vi "computername.vi"(2 "error in (no error)":errorcluster, 3 "value":string="ComputerName", 4 "subkey":string="System\\CurrentControlSet\\Control\\ComputerName\\ComputerName", 5 "root key (HKEY_LOCAL_MACHINE)":T1=enum."HKEY_LOCAL_MACHINE") -> (0 "error out":errorcluster, 1 "String/Binary data":string)   [LabVIEW 2018]
doc: "This example program uses the Registry VIs in LabVIEW to access the Windows registry and obtain the computer name."
uses:
  <vilib>/registry/registry.llb/Registry RtKey.ctl
  <vilib>/registry/registry.llb/Read Registry Value Simple STR.vi
panel:
  # "This example program uses the Registry VIs in LabVIEW to access the Windows registry and obtain the computer name.\n\nTo Run the program, click on the Run arrow. The computer name will be shown in the 'String/Binary data' string indicator."
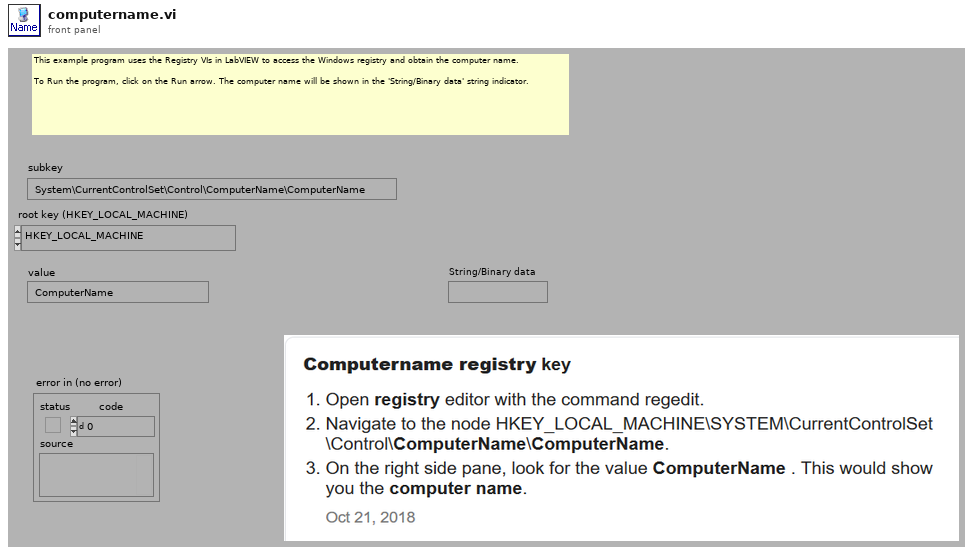
[diagram p1: front panel]
types:
  T1 = typedef "Registry RtKey.ctl" = enum32{"HKEY_CLASSES_ROOT", "HKEY_CURRENT_USER", "HKEY_LOCAL_MACHINE", "HKEY_USERS", "HKEY_PERFORMANCE_DATA", "HKEY_CURRENT_CONFIG", "HKEY_DYN_DATA"}
  T2 = typedef "Registry refnum.ctl" = refnum<k1>
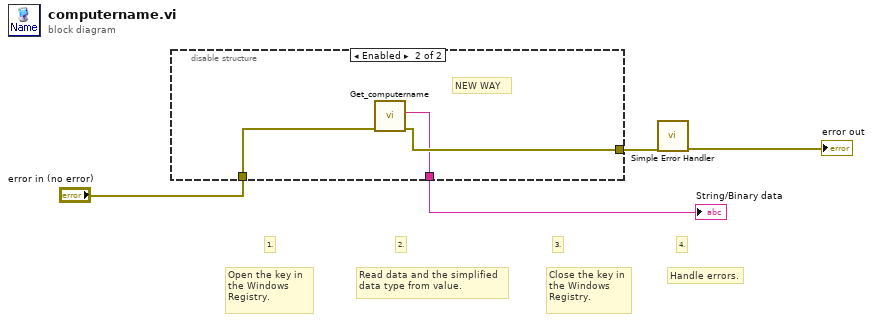
[diagram p0: block diagram]
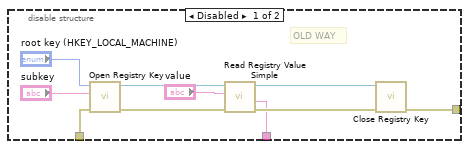
[diagram p2: hidden frame]
diagram:
  # "Handle errors."
  # "4."
  # "Close the key in\nthe Windows\nRegistry."
  # "3."
  # "Read data and the simplified\ndata type from value."
  # "2."
  # "Open the key in \nthe Windows\nRegistry."
  # "1."
  n1 = disable-structure shown="Enabled" {
    disable-tunnel: [w10 w16] -> w4
    disable-tunnel: [w8 w15] -> w3
    disable-tunnel: "error in (no error)" -> [w5 w17]
    frame Disabled {
      # "OLD WAY"
      n2 = call <vilib>:"Open Registry Key.vi"("error in (no error)"=w5, "subkey"="subkey", "root key (HKEY_LOCAL_MACHINE)"="root key (HKEY_LOCAL_MACHINE)") -> ("error out"=w14:errorcluster, "refnum out"=w13:T2)  [unwired: 7 in]
      n3 = call-poly <vilib>:"Read Registry Value Simple.vi"("error in (no error)"=w14, "value"="value", "refnum"=w13) -> ("error out"=w12:errorcluster, "String/Binary data"=w8:string, "refnum out"=w11:T2)  [unwired: 3 in, 1 out]
      n4 = call <vilib>:"Close Registry Key.vi"("error in (no error)"=w12, "refnum"=w11) -> ("error out"=w10:errorcluster)  [unwired: 5 in]
    }
    frame Enabled {
      # "NEW WAY"
      n5 = call "Get_computername.vi"("error in (no error)"=w17) -> ("error out"=w16:errorcluster, "Computer Name"=w15:string)  [unwired: 9 in]
    }
  }
  "String/Binary data" <- w3
  n6 = call <vilib>:"Simple Error Handler.vi"("error in (no error)"=w4) -> ("error out"=→"error out":errorcluster)  [unwired: 4 in, 4 out]
